vi "Test_getEvent_simulationMode.vi"(8 "error in (no error)":errorcluster, 11 "logevent_simulationMode_Ctl":T1) -> (0 "error out":errorcluster, 2 "function return":i32, 3 "logevent_simulationMode_Ctl out":T1)   [LabVIEW 2016, in "SALLV_Test.lvlib"]
doc: "int Test_shm_getEvent_simulationModeLV(Test_logevent_simulationModeLV *logevent_simulationMode_Ctl );"
uses:
  SALLV_Test.lvlib
  DataTypes/logevent_simulationMode.ctl
  SALLV_Test.so
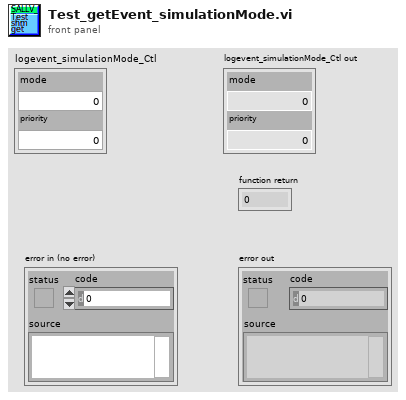
[diagram p1: front panel]
types:
  T1 = typedef "SALLV_Test.lvlib/logevent_simulationMode.ctl" = cluster{"mode":i32, "priority":i32}
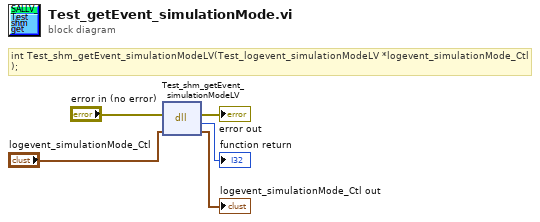
[diagram p0: block diagram]
diagram:
  # "int Test_shm_getEvent_simulationModeLV(Test_logevent_simulationModeLV *logevent_simulationMode_Ctl );"
  n1 = dll-call lib="home/ccontaxis/Code/SALLV_Test/SALLV_Test.*" fn="Test_shm_getEvent_simulationModeLV"(error in="error in (no error)", "logevent_simulationMode_Ctl"="logevent_simulationMode_Ctl") -> (error out=→"error out":errorcluster, →"function return":i32, "logevent_simulationMode_Ctl"=→"logevent_simulationMode_Ctl out":T1)  [unwired: 2 in, 1 out]
